vi "UUT Test.vi"(8 "error in (no error)":errorcluster, 11 "PLC_Module in":refnum<class "PLC_Module.lvclass">) -> (0 "error out":errorcluster, 3 "PLC_Module out":refnum<class "PLC_Module.lvclass">)   [LabVIEW 2025, in "PLC_Module.lvlib" / "PLC_Module.lvclass"]
uses:
  PLC_Module.lvclass
  PLC_Module.lvclass/PLC_Module.ctl
  40f895c0-9560-4bb7-a7a3-c0324d7c3b54.vi
  Read Configuration.vi
  <vilib>/JDP Science/JSONtext/JSON text to Variant.vi
  <vilib>/JDP Science/JSONtext/LVClass Serializer/JSONtext LVClass Serializer.lvclass
  <userlib>/_OpenG.lib/boolean/boolean.llb/openg_boolean__ogtk.lvlib
  <vilib>/Test Bench Framework/UUT Test(Context).vi
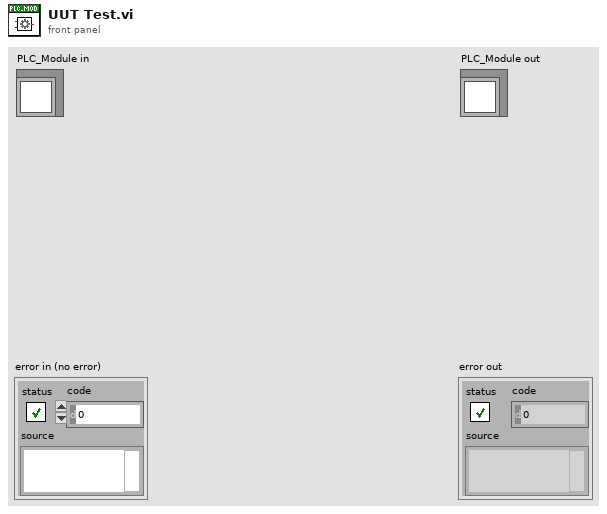
[diagram p1: front panel]
types:
  T1 = typedef "PLC_Module.lvlib/PLC_Module.lvclass/PLC_Data_Config.ctl" = map{string, cluster{"Config":T2, "Get Value":string, "Set Value":string}}
  T2 = typedef "PLC_Module.lvlib/PLC_Module.lvclass/PLC_Data.ctl" = cluster{"Address":string, "Direction":enum16{"PC->PLC", "PLC->PC"}, "DataType":T3, "Description":string}
  T3 = typedef "PLC_Module.lvlib/PLC_Module.lvclass/PLC_Data_Type.ctl" = enum16{"Boolean", "Single Float", "U8", "U32", "U32_Array", "String"}
  T4 = cluster{"Config":T2, "Get Value":string, "Set Value":string}
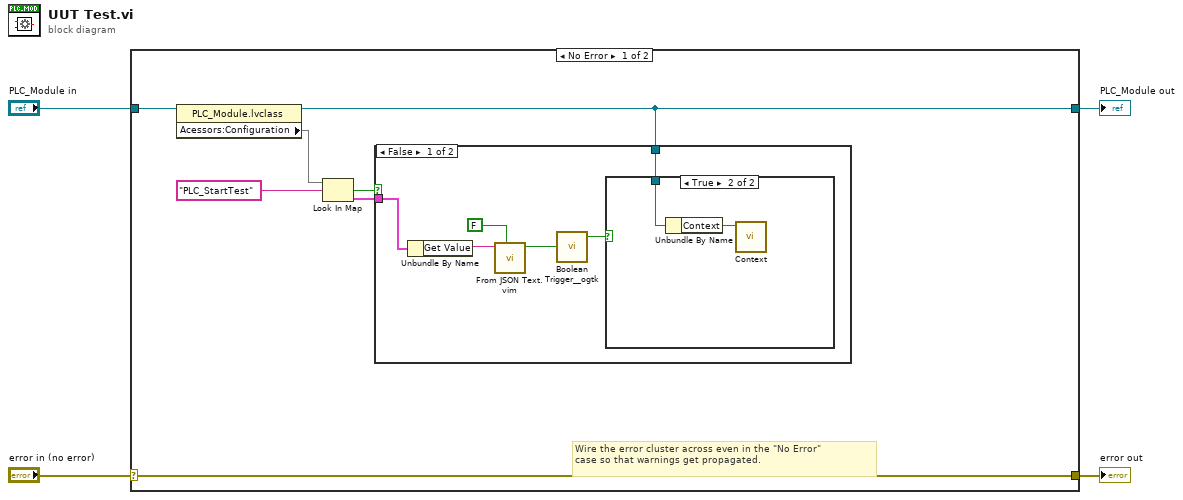
[diagram p0: block diagram]
diagram:
  n1 = case shown="No Error" "error in (no error)" {
    selector: "error in (no error)" -> [w11 w21]
    tunnel: [w11 w21] -> w3
    tunnel: [w9 w20] -> w1
    tunnel: "PLC_Module in" -> [w10 w20]
    frame No Error {
      # "Wire the error cluster across even in the \"No Error\"\ncase so that warnings get propagated."
      n2 = property class="PLC_Module.lvclass"(reference=w10) -> (reference out=w9:refnum<class "PLC_Module.lvclass">, "Acessors:Configuration"=w8:T1)  [unwired: 1 in, 1 out]
      n3 = Look In Map(map=w8, key="PLC_StartTest") -> (key not found?=w5:bool, value=w6:T4)  [unwired: 1 in]
      n4 = case shown="False" w5 {
        tunnel: w9 -> [w17 _]
        tunnel: w6 -> [w16 _]
        frame False {
          n5 = Unbundle By Name(w16) -> ("Get Value"=w15:string)
          n6 = call "From JSON Text.vim"("Data Type and Default Value"=FALSE, "JSON"=w15) -> ("Data out"=w13:bool)  [unwired: 8 in, 1 out]
          n7 = call <userlib>:"Boolean Trigger__ogtk.vi"("Boolean Input"=w13) -> ("Rising Edge"=w12:bool)  [unwired: 1 in, 1 out]
          n8 = case shown="True" w12 {
            tunnel: w17 -> [_ w18]
            frame False {
            }
            frame True {
              n9 = Unbundle By Name(w18) -> ("Context"=w19:refnum<vi>)
              n10 = call-poly <vilib>:"Context.vi"("Context"=w19) -> ()  [unwired: 10 in, 1 out]
            }
          }
        }
        frame True {
        }
      }
    }
    frame Error {
    }
  }
  "error out" <- w3
  "PLC_Module out" <- w1
